vi "A2v.vi"() -> ()   [LabVIEW 2020]
panel:
  out "Temperature History":cluster{dbl, "Temperature":dbl}(graph)
  in  "Power":bool
  # "ON"
  # "OFF"
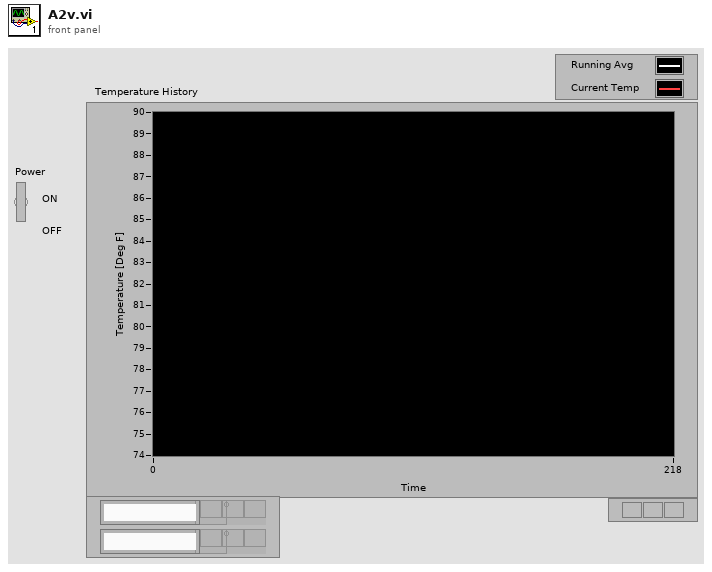
[diagram p1: front panel]
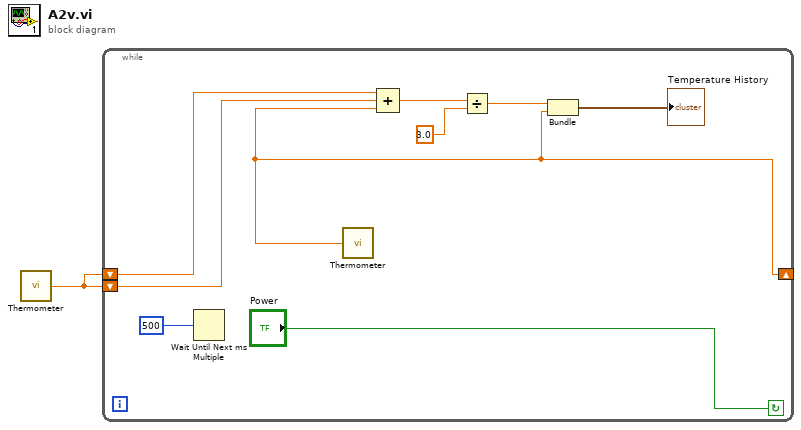
[diagram p0: block diagram]
diagram:
  n1 = call "Thermometer.vi"() -> ("Temperature"=w1:dbl)  [unwired: 1 in]
  n2 = while {
    shift-right: [w4] -> _
    shift-left: w1 -> [w7]
    shift-left: w1 -> [w6]
    stop <- "Power" continue-if-true
    n3 = Wait Until Next ms Multiple(millisecond multiple=u32 500) -> ()  [unwired: 1 out]
    n4 = call "Thermometer.vi"() -> ("Temperature"=w4:dbl)  [unwired: 1 in]
    n5 = Compound Arithmetic op=ADD(w7, w6, w4) -> (w8:dbl)
    n6 = Divide(x=w8, y=3.0) -> (x/y=w5:dbl)
    n7 = Bundle(w5, "Temperature"=w4) -> (→"Temperature History":cluster{dbl, "Temperature":dbl})  [unwired: 1 in]
  }
